vi "_TangoSubscribeMultipleAttributeEvents.vi"(2 "error in":errorcluster, 3 "events types":T3[](array[typedef])=[enum."UNKNOWN_EVENT", enum."UNKNOWN_EVENT"], 4 "events sources":string[][](array[string])=[["", ""], ["", ""]], 5 "attribute event ref.":T1) -> (0 "error out":errorcluster, 1 "subscribed events":T2={"events sources"=[["", ""], ["", ""], ["", ""]], "events types"=[enum."UNKNOWN_EVENT", enum."UNKNOWN_EVENT"]})   [LabVIEW 2014, in "tango.lvlib"]
uses:
  tango.lvlib
  Private VIs/Events/_EventType.ctl
  Common VIs/Typedefs/_AttributeEventRef.ctl
  Common VIs/Typedefs/_AttributeValue_t.ctl
  Common VIs/Typedefs/_AttributeQuality_t.ctl
  Common VIs/Typedefs/_AttributeDataType_t.ctl
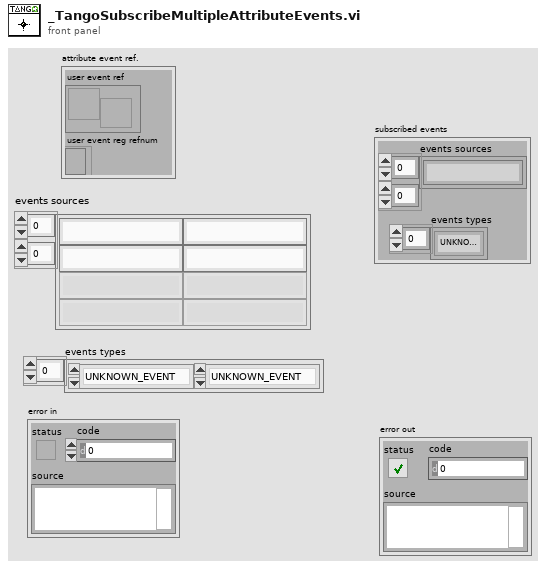
[diagram p1: front panel]
types:
  T1 = typedef "tango.lvlib/_AttributeEventRef.ctl" = cluster{"user event ref":refnum<user-event>, "user event reg refnum":refnum<event-registration>}
  T2 = cluster{"events sources":string[][], "events types":enum32{"CHANGE_EVENT", "DEPRECATED_QUALITY_EVENT", "PERIODIC_EVENT", "ARCHIVE_EVENT", "USER_EVENT", "ATTRIBUTE_CONF_EVENT", "DATA_READY_EVENT", "INTERFACE_CHANGE_EVENT", "UNKNOWN_EVENT"}[]}
  T3 = typedef "tango.lvlib/_EventType.ctl" = enum32{"CHANGE_EVENT", "DEPRECATED_QUALITY_EVENT", "PERIODIC_EVENT", "ARCHIVE_EVENT", "USER_EVENT", "ATTRIBUTE_CONF_EVENT", "DATA_READY_EVENT", "INTERFACE_CHANGE_EVENT", "UNKNOWN_EVENT"}
  T4 = cluster{"events sources":string[][], "events types":T3[]}
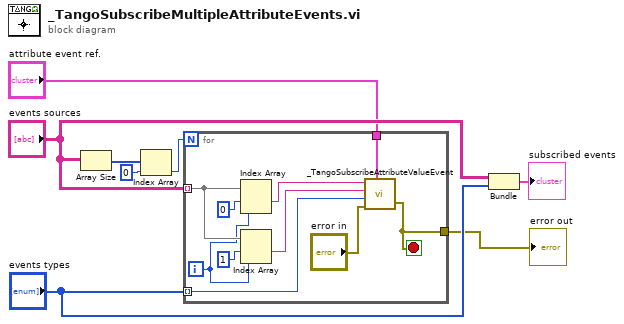
[diagram p0: block diagram]
diagram:
  n1 = Array Size(array="events sources") -> (size(s)=w7:i32[])
  n2 = Index Array(array=w7, index=0) -> (element=w6:i32)
  n3 = for {
    N: w6 -> [_]
    tunnel: "events sources" -> [w18] mode=indexing
    tunnel: "events types" -> [w15] mode=indexing
    tunnel: [w13] -> w3
    tunnel: "attribute event ref." -> [w9]
    i -> [w10]
    stop <- w13 stop-if-true
    n4 = Index Array(array=w18, index #1=0 ("index"), index #2=w10) -> (element #1=w17:string)  [unwired: 1 out]
    n5 = Index Array(array=w18, index #1=1 ("index"), index #2=w10) -> (element #1=w16:string)  [unwired: 1 out]
    n6 = call "_TangoSubscribeAttributeValueEvent.vi"("device name"=w17, "attribute name"=w16, "tango event type"=w15, "error in"="error in", "attribute event ref."=w9) -> ("error out"=w13:errorcluster)  [unwired: 1 out]
  }
  "error out" <- w3
  n7 = Bundle("events sources"="events sources", "events types"="events types") -> (→"subscribed events":T4)  [unwired: 1 in]
